vi "LJStreamM command response read channels.vi"(0 "Handle In":i32, 5 "# Channels":i32, 7 "Disable Scaling":bool, 9 "Channel Setup In":T1={"Name"=["AIN0", "AIN1", "AIN2", "AIN3", "AIN4", "AIN5", "AIN6", "AIN7", "AIN8", "AIN9", "AIN10", "AIN11", "AIN12", "AIN13", "AIN14", "AIN15"], "", "Scaling Equation"=["y=a", "y=b", "y=c", "y=d", "y=e", "y=f", "y=g", "y=h", "y=i", "y=j", "y=k", "y=l", "y=m", "y=n", "y=o", "y=p"], "", "Graph?"=[TRUE, TRUE, TRUE, TRUE, FALSE, FALSE, FALSE, FALSE, FALSE, FALSE, FALSE, FALSE, FALSE, FALSE, FALSE, FALSE]}, 11 "Error In":errorcluster) -> (4 "Handle Out":i32, 6 "Raw Data":dbl[](array[numeric]), 8 "Scaled Data":dbl[](array[numeric]), 13 "Error Message":string="No Error", 14 "Error Message Status":bool, 15 "(LJM) Error Out":errorcluster)   [LabVIEW 2026]
uses:
  Common Logger Controls/Channel Setup.ctl
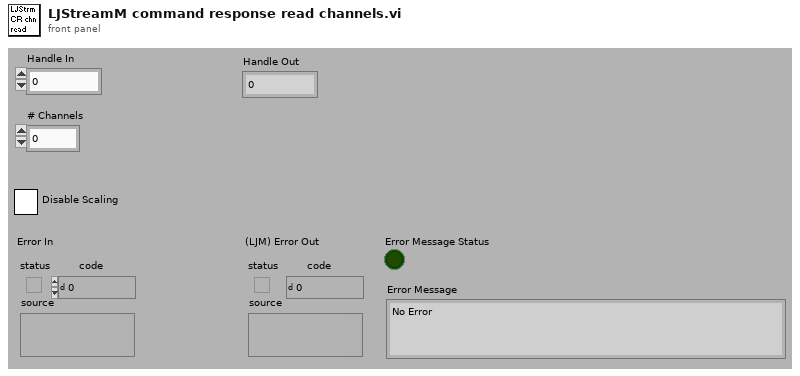
[diagram p1: front panel]
types:
  T1 = typedef "Channel Setup.ctl" = cluster{"Name":string[], string, "Scaling Equation":string[], string, "Graph?":bool[]}
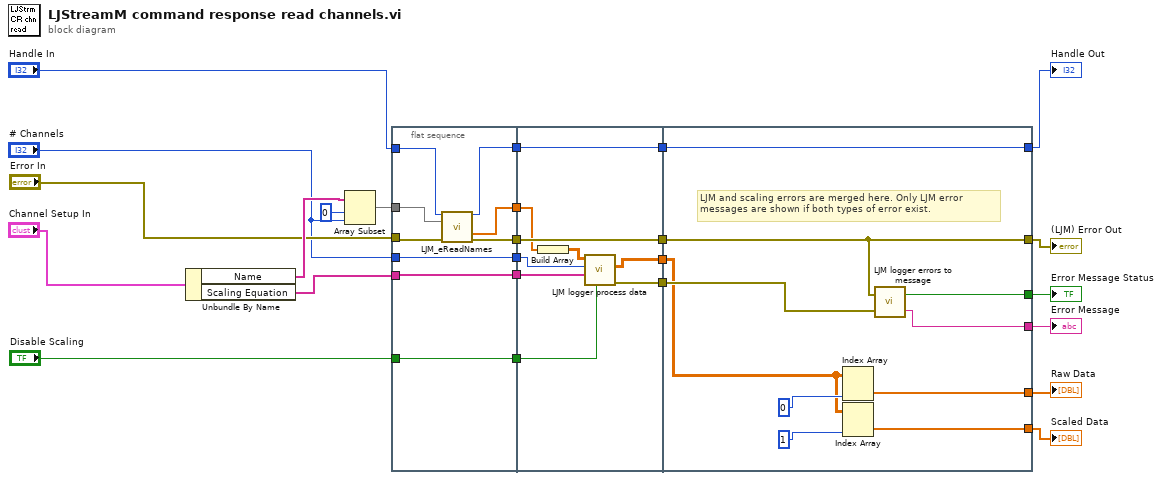
[diagram p0: block diagram]
diagram:
  n1 = Unbundle By Name("Channel Setup In") -> ("Name"=w23:string[], "Scaling Equation"=w13:string[])
  n2 = Array Subset(array=w23, index=0 ("Array Index"), length="# Channels") -> (w24:string[])
  n3 = flat-sequence {
    tunnel: w24 -> [w34]
    tunnel: "Error In" -> [w32]
    tunnel: "Handle In" -> [w31]
    tunnel: [w33] -> w19
    tunnel: [w30] -> w18
    tunnel: [w29] -> w17
    tunnel: w13 -> [w28]
    tunnel: [w28] -> w14
    tunnel: [w27] -> w9
    tunnel: "# Channels" -> [w27]
    tunnel: "Disable Scaling" -> [w26]
    tunnel: [w26] -> w1
    tunnel: w19 -> [w36]
    tunnel: w18 -> [w43]
    tunnel: w17 -> [w42]
    tunnel: [w43] -> w16
    tunnel: [w42] -> w15
    tunnel: w14 -> [w39]
    tunnel: w9 -> [w38]
    tunnel: [w41] -> w4
    tunnel: [w40] -> w3
    tunnel: w1 -> [w35]
    tunnel: [w48] -> w10
    tunnel: [w53] -> w20
    tunnel: w16 -> [w53]
    tunnel: w15 -> [w48]
    tunnel: [w50] -> w12
    tunnel: [w49] -> w11
    tunnel: [w47] -> w6
    tunnel: [w46] -> w5
    tunnel: w4 -> [w45]
    tunnel: w3 -> [w44]
    frame #0 {
      n4 = call "LJM_eReadNames.vi"("Handle In"=w31, "aNames"=w34, "error in"=w32) -> ("Handle Out"=w30:i32, "aValuesOut"=w33:dbl[], "error out"=w29:errorcluster)  [unwired: 9 in, 1 out]
    }
    frame #1 {
      n5 = Build Array(w36) -> (w37:dbl[][])
      n6 = call "LJM logger process data.vi"("Disable Scaling"=w35, "Scaling Equation"=w39, "# Channels"=w38, "Voltages"=w37) -> ("error out"=w41:errorcluster, "Volts,Scaled Averages"=w40:dbl[][])  [unwired: 5 in, 1 out]
    }
    frame #2 {
      # "LJM and scaling errors are merged here. Only LJM error messages are shown if both types of error exist."
      n7 = Index Array(array=w44, index (col)=0 ("Disabled Index (col)")) -> (element=w47:dbl[])  [unwired: 1 in]
      n8 = Index Array(array=w44, index (col)=1 ("Disabled Index (col)")) -> (element=w46:dbl[])  [unwired: 1 in]
      n9 = call "LJM logger errors to message.vi"("Scaling Error"=w45, "LJM Error"=w48) -> ("Error Message"=w49:string, "status"=w50:bool)
    }
  }
  "Handle Out" <- w20
  "(LJM) Error Out" <- w10
  "Error Message" <- w11
  "Error Message Status" <- w12
  "Raw Data" <- w6
  "Scaled Data" <- w5
